vi "CheckAddsOnDeploy.vi"(5 "System Definition Dir":path, 6 "IP address":string, 7 "Details Ref":refnum<vi>, 8 "error in (no error)":errorcluster, 10 "ftp session":T2, 11 "Device Item Ref in":T1 format="%.0x") -> (0 "error out":errorcluster, 2 "ftp session out":T2, 3 "Device Item Ref out":T1 format="%.0x")   [LabVIEW 2010, in "RefMem PtByPt Custom Device.lvlib"]
uses:
  RefMem PtByPt Custom Device.lvlib
  <vilib>/addons/internet/ftp/ftp0.llb/FTP Session.ctl
  <vilib>/NI Veristand/Custom Device API/Custom Device Item Ref.ctl
  NationalInstruments.VeriStand.SystemStorage
  Controls/Global.vi
  <vilib>/NI Veristand/Custom Device API/Custom Device API.lvlib
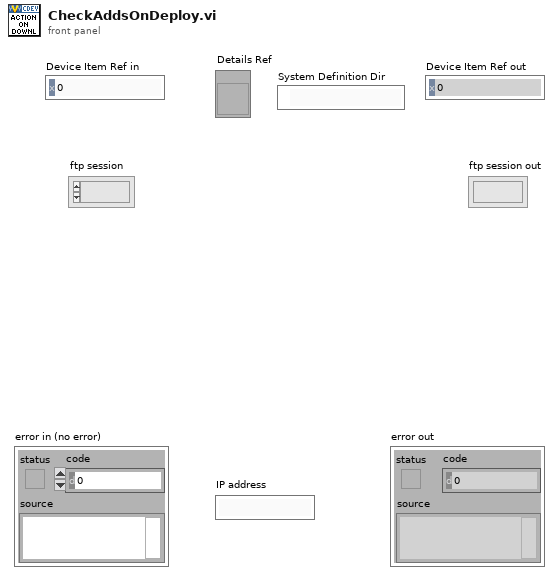
[diagram p1: front panel]
types:
  T1 = typedef "Custom Device API.lvlib/Custom Device Item Ref.ctl" = u64
  T2 = typedef "FTP Session.ctl" = refnum<k1>
  T3 = typedef "Custom Device API.lvlib/Custom Device Pointer.ctl" = refnum<k24>
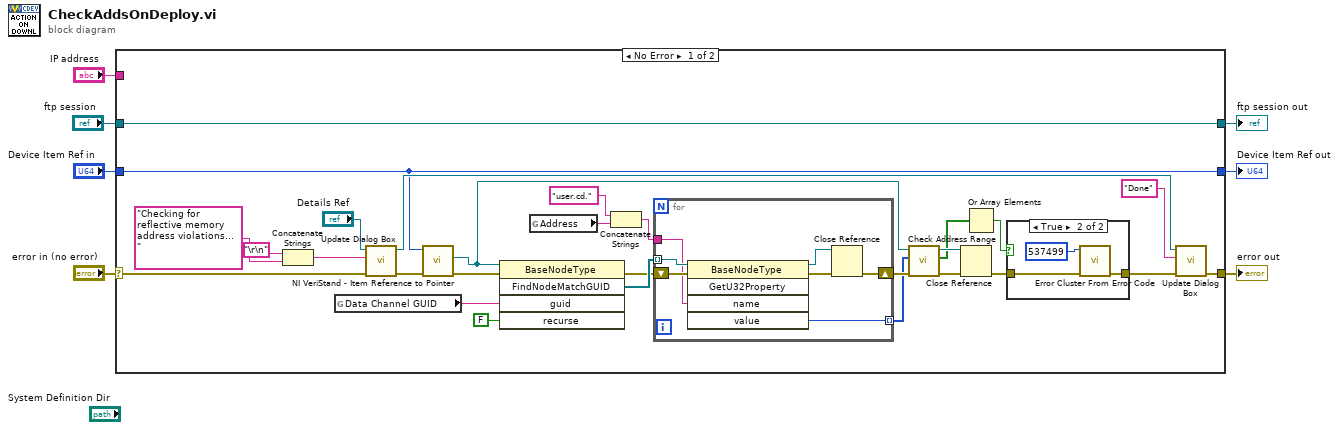
[diagram p0: block diagram]
diagram:
  n1 = case shown="No Error" "error in (no error)" {
    selector: "error in (no error)" -> [w17 w49]
    tunnel: [w31 w49] -> w6
    tunnel: "ftp session" -> [w35 w48]
    tunnel: [w35 w48] -> w4
    tunnel: "Device Item Ref in" -> [w27 w47]
    tunnel: [w27 w47] -> w2
    tunnel: "IP address" -> [_ _]
    frame No Error {
      n2 = Concatenate Strings("\r\n", "Checking for reflective memory address violations... " ("string")) -> (w32:string)
      n3 = global read "Global.vi" "Data Channel GUID"() -> (w24:string)
      n4 = call "Update Dialog Box.vi"("error in (no error)"=w17, "Text to add"=w32, "Details Ref in"="Details Ref") -> ("error out"=w18:errorcluster, "Details Ref out"=w30:refnum<vi>)  [unwired: 7 in]
      n5 = call <vilib>:"NI VeriStand - Item Reference to Pointer.vi"("error in (no error)"=w18, "Item Ref in"=w27) -> ("error out"=w26:errorcluster, "Node Pointer"=w14:T3)  [unwired: 6 in, 2 out]
      n6 = invoke class="BaseNodeType" method="FindNodeMatchGUID"(reference=w14, error in=w26, "guid"=w24, "recurse"=FALSE) -> (error out=w22:errorcluster, "FindNodeMatchGUID"=w23:refnum<k24>[])  [unwired: 1 in, 3 out]
      n7 = global read "Global.vi" "Address"() -> (w21:string)
      n8 = Concatenate Strings("user.cd." ("string"), w21) -> (w19:string)
      n9 = for {
        tunnel: w23 -> [w45] mode=indexing
        shift-right: [w42] -> w15
        shift-left: w22 -> [w46]
        tunnel: w19 -> [w44]
        tunnel: [w40] -> w13 mode=indexing
        n10 = invoke class="BaseNodeType" method="GetU32Property"(reference=w45, error in=w46, "name"=w44) -> (reference out=w41:refnum<k24>, error out=w43:errorcluster, "value"=w40:u32)  [unwired: 2 in, 2 out]
        n11 = Close Reference(reference=w41, error in (no error)=w43) -> (error out=w42:errorcluster)
      }
      n12 = call "Check Address Range.vi"("error in (no error)"=w15, "Addresses"=w13, "Node Pointer In"=w14) -> ("error out"=w12:errorcluster, "Inside NIVS Range"=w9:bool[], "Node Pointer dup"=w10:T3)  [unwired: 6 in]
      n13 = Close Reference(reference=w10, error in (no error)=w12) -> (error out=w11:errorcluster)
      n14 = Or Array Elements(Boolean array=w9) -> (logical OR=w8:bool)
      n15 = case shown="True" w8 {
        tunnel: w11 -> [w36 w38]
        tunnel: [w36 w37] -> w16
        frame False {
        }
        frame True {
          n16 = call <vilib>:"Error Cluster From Error Code.vi"("error in (no error)"=w38, "error code (0)"=537499) -> ("error out"=w37:errorcluster)  [unwired: 7 in]
        }
      }
      n17 = call "Update Dialog Box.vi"("error in (no error)"=w16, "Text to add"="Done" ("string"), "Details Ref in"=w30) -> ("error out"=w31:errorcluster)  [unwired: 7 in, 1 out]
    }
    frame Error {
    }
  }
  "error out" <- w6
  "ftp session out" <- w4
  "Device Item Ref out" <- w2
